vi "CanStatusShow.vi"(10 "DevIndex":u32, 11 "DevType":u16) -> ()   [LabVIEW 2011]
doc: "ID=0x6005"
panel:
  out "label2":string="寄存器信息"
  in  "OK":bool
  out "regTECounter":u8 caption="Send error register:" format="0x%02x"
  out "regRECounter":u8 caption="Receiving error register:" format="0x%02x"
  out "regEWLimit":u8 caption="Error warning limit register:" format="0x%02x"
  out "regECCapture":u8 caption="Error register:" format="0x%02x"
  out "regALCapture":u8 caption="Arbitration lost register:" format="0x%02x"
  out "regStatus":u8 caption="State Register：" format="0x%02x"
  out "regMode":u8 caption="Mode Register:" format="0x%02x"
  out "ErrInterrupt":u8 caption="Interrupt record：" format="0x%02x"
  in  "Update":bool
  in  "udtTime":i32=1 min=1 max=100 format="%d s"
  in  "Auto":bool
  in  "channel":u16(ring) caption="Channel:" items=["Ch1", "Ch2"]
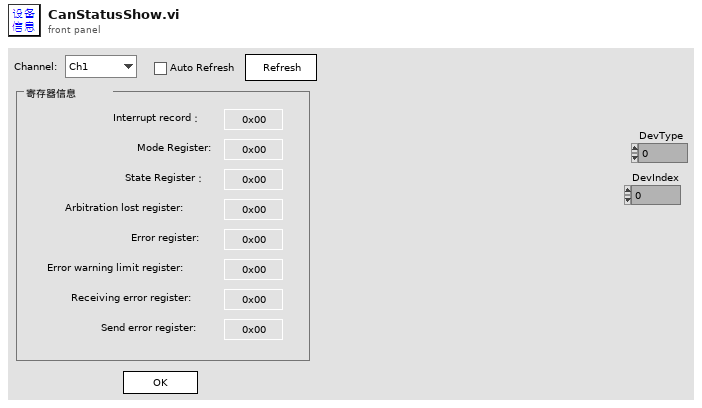
[diagram p1: front panel]
types:
  T1 = cluster{"ErrInterrupt":u8, "regMode":u8, "regStatus":u8, "regALCapture":u8, "regECCapture":u8, "regEWLimit":u8, "regRECounter":u8, "regTECounter":u8, "Reserved":u32}
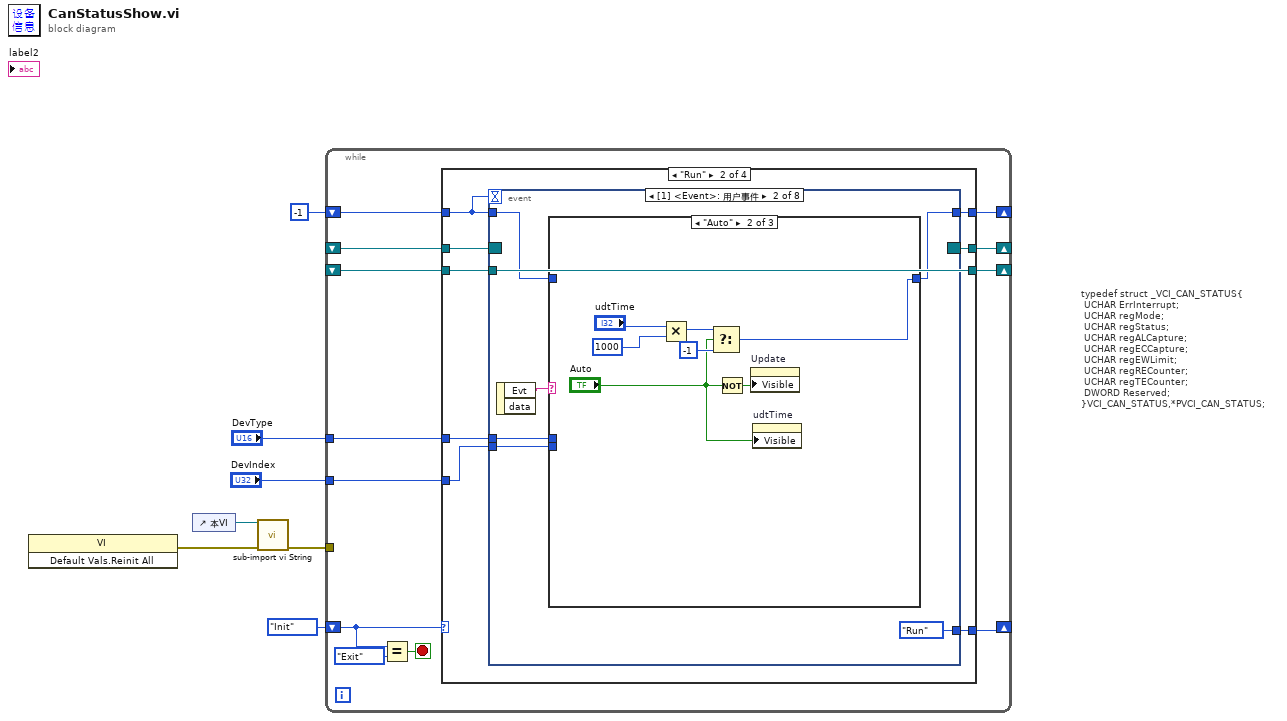
[diagram p0: block diagram]
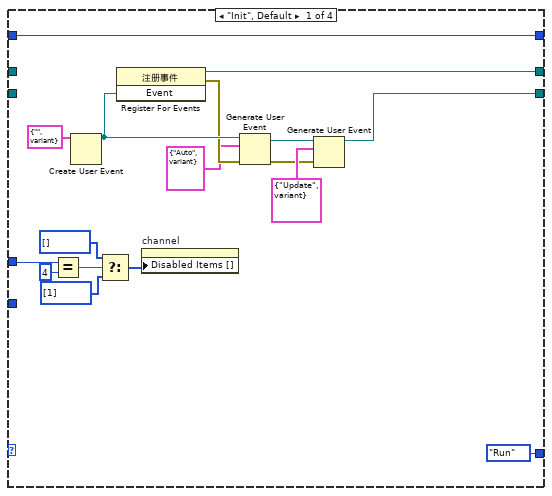
[diagram p2: hidden frame]
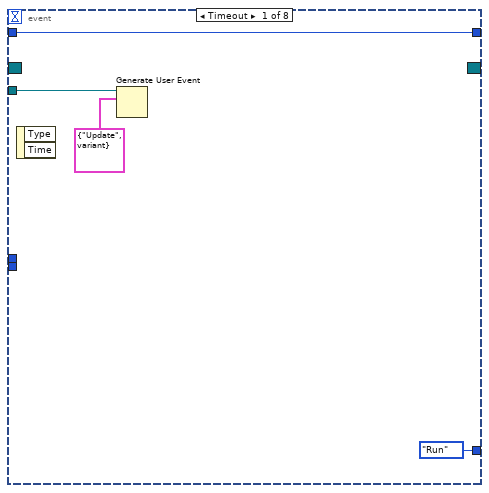
[diagram p3: hidden frame]
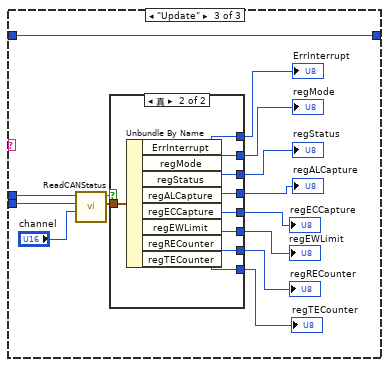
[diagram p5: hidden frame]
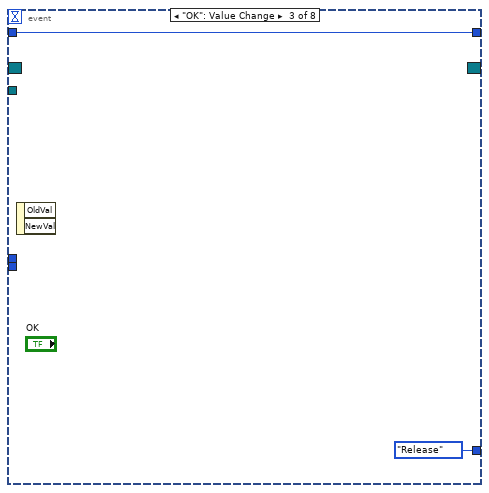
[diagram p7: hidden frame]
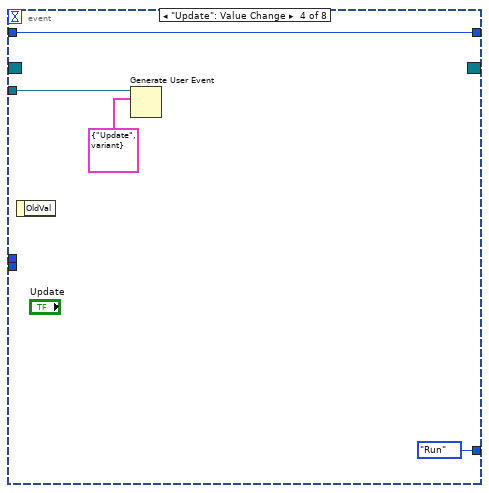
[diagram p8: hidden frame]
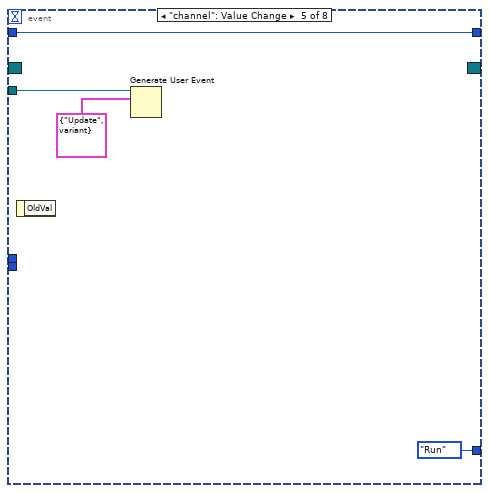
[diagram p9: hidden frame]
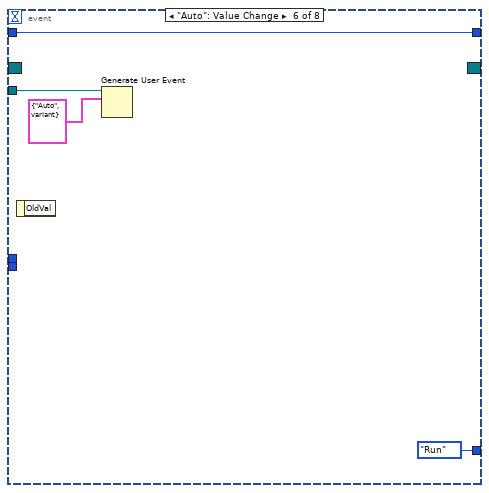
[diagram p10: hidden frame]
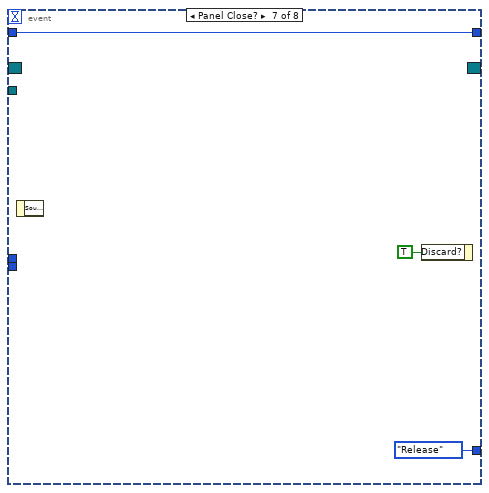
[diagram p11: hidden frame]
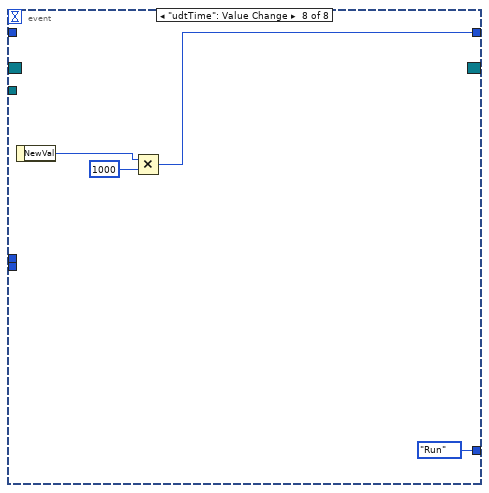
[diagram p12: hidden frame]
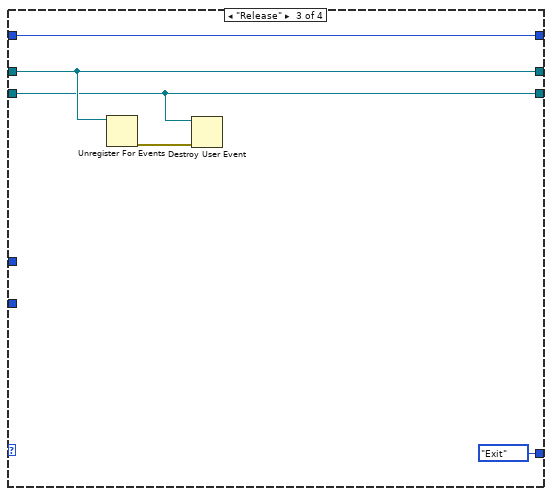
[diagram p13: hidden frame]
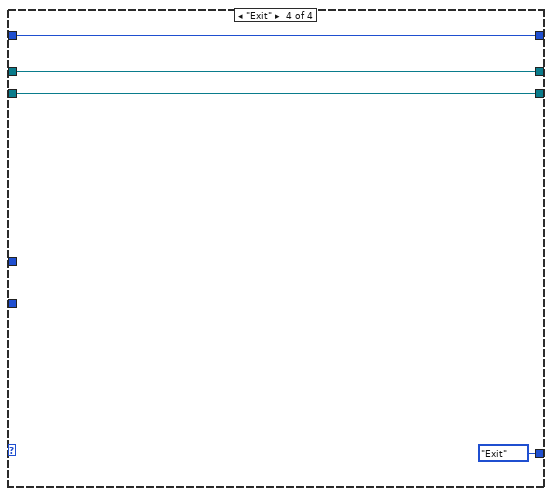
[diagram p14: hidden frame]
diagram:
  # "typedef struct _VCI_CAN_STATUS{\n\tUCHAR\tErrInterrupt;\n\tUCHAR\tregMode;\n\tUCHAR\tregStatus;\n\tUCHAR\tregALCapture;\n\tUCHAR\tregECCapture; \n\tUCHAR\tregEWLimit;\n\tUCHAR\tregRECounter; \n\tUCHAR\tregTECounter;\n\tDWORD\tReserved;\n}VCI_CAN_STATUS,*PVCI_CAN_STATUS;"
  n1 = invoke class="VI" method="Default Vals.Reinit All"() -> (error out=w1:errorcluster)  [unwired: 3 in, 2 out]
  n2 = control-ref of="本VI"() -> (w3:refnum<vi>)
  n3 = call "sub-import vi String.vi"("error in (no error)"=w1, "vi ref"=w3) -> ("error out"=w2:errorcluster)  [unwired: 9 in]
  n4 = while {
    shift-right: [w16] -> _
    shift-left: enum16{"Init", "Run", "Release", "Exit"}."Init" -> [w19]
    shift-right: [w15] -> _
    shift-left: _ -> [w14]
    tunnel: "DevType" -> [w13]
    tunnel: "DevIndex" -> [w12]
    shift-right: [w11] -> _
    shift-left: _ -> [w10]
    shift-right: [w8] -> _
    shift-left: -1 -> [w9]
    tunnel: w2 -> [_]
    stop <- w17 stop-if-true
    n5 = Equal?(x=w19, y=enum16{"Init", "Run", "Release", "Exit"}."Exit") -> (x = y?=w17:bool)
    n6 = case shown="\"Run\"" w19 {
      tunnel: [enum16{"Init", "Run", "Release", "Exit"}."Run" w44 enum16{"Init", "Run", "Release", "Exit"}."Exit" enum16{"Init", "Run", "Release", "Exit"}."Exit"] -> w16
      tunnel: [w34 w42 w110 w115] -> w15
      tunnel: w14 -> [_ w43 w110 w115]
      tunnel: w13 -> [w30 w38 _ _]
      tunnel: w12 -> [_ w37 _ _]
      tunnel: [w21 w41 w109 w114] -> w11
      tunnel: w10 -> [_ w41 w109 w114]
      tunnel: w9 -> [w20 w40 w111 w113]
      tunnel: [w20 w39 w111 w113] -> w8
      frame "Init", Default {
        n7 = Equal?(x=w30, y=u16 4) -> (x = y?=w28:bool)
        n8 = Create User Event(user event datatype=cluster{"Evt":string, "data":variant} {"Evt"="", "data"=variant} ("Event")) -> (user event=w33:refnum<user-event>)  [unwired: 1 in, 1 out]
        n9 = Select(t=i32[] [] ("禁用项[]"), s=w28, f=i32[] [1] ("禁用项[]")) -> (s? t:f=w25:i32[])
        n10 = register-events(w33) -> (reference out=w34:refnum<event-registration>, error out=w32:errorcluster)  [unwired: 2 in]
        n11 = property on="channel" class="Ring (严格)"("Disabled Items []"=w25) -> ()  [unwired: 2 in, 2 out]
        n12 = Generate User Event(user event=w33, event data cluster=cluster{"Evt":string, "data":variant} {"Evt"="Auto", "data"=variant} ("事件数据"), error in=w32) -> (user event out=w23:refnum<user-event>, error out=w22:errorcluster)
        n13 = Generate User Event(user event=w23, event data cluster=cluster{"Evt":string, "data":variant} {"Evt"="Update", "data"=variant} ("事件数据"), error in=w22) -> (user event out=w21:refnum<user-event>)  [unwired: 1 out]
      }
      frame "Run" {
        n14 = event shown="[1] <Event>: 用户事件" {
          selector: w43 -> [_ _ _ _ _ _ _ _]
          dyn-events: [_ _ _ _ _ _ _ _] -> w42
          timeout: w40 -> [_ _ _ _ _ _ _ _]
          tunnel: [enum16{"Init", "Run", "Release", "Exit"}."Run" enum16{"Init", "Run", "Release", "Exit"}."Run" enum16{"Init", "Run", "Release", "Exit"}."Release" enum16{"Init", "Run", "Release", "Exit"}."Run" enum16{"Init", "Run", "Release", "Exit"}."Run" enum16{"Init", "Run", "Release", "Exit"}."Run" enum16{"Init", "Run", "Release", "Exit"}."Release" enum16{"Init", "Run", "Release", "Exit"}."Run"] -> w44
          tunnel: w41 -> [w45 _ _ w88 w92 w98 _ _]
          tunnel: w40 -> [w47 w52 w86 w90 w94 w97 w100 _]
          tunnel: [w47 w51 w86 w90 w94 w97 w100 w103] -> w39
          tunnel: w38 -> [_ w50 _ _ _ _ _ _]
          tunnel: w37 -> [_ w49 _ _ _ _ _ _]
          event Timeout {
            n15 = event-data() -> ()  [unwired: 1 in, 2 out]
            n16 = Generate User Event(user event=w45, event data cluster=cluster{"Evt":string, "data":variant} {"Evt"="Update", "data"=variant} ("事件数据")) -> ()  [unwired: 1 in, 2 out]
          }
          event User Event {
            n17 = event-data() -> ("Evt"=w53:string)  [unwired: 1 in, 1 out]
            n18 = case shown="\"Auto\"" w53 {
              tunnel: w52 -> [w55 _ w76]
              tunnel: [w55 w59 w76] -> w51
              tunnel: w50 -> [_ _ w75]
              tunnel: w49 -> [_ _ w74]
              frame "假", Default {
              }
              frame "Auto" {
                n19 = Multiply(x="udtTime", y=1000) -> (x*y=w60:i32)
                n20 = Select(t=w60, s="Auto", f=-1) -> (s? t:f=w59:i32)
                n21 = Not(x="Auto") -> (.not. x?=w57:bool)
                n22 = property on="Update" class="Bool"("Visible"=w57) -> ()  [unwired: 2 in, 2 out]
                n23 = property on="udtTime" class="DigNum (严格)"("Visible"="Auto") -> ()  [unwired: 2 in, 2 out]
              }
              frame "Update" {
                n24 = call "ReadCANStatus.vi"("CANInd"="channel", "DeciceInd"=w74, "DeviceType"=w75) -> ("VCI_CAN_STATUS"=w71:T1, "Valid"=w72:bool)  [unwired: 6 in, 1 out]
                n25 = case shown="真" w72 {
                  tunnel: w71 -> [_ w85]
                  tunnel: [_ w84] -> w70
                  tunnel: [_ w83] -> w69
                  tunnel: [_ w82] -> w68
                  tunnel: [_ w81] -> w67
                  tunnel: [_ w80] -> w66
                  tunnel: [_ w79] -> w65
                  tunnel: [_ w78] -> w64
                  tunnel: [_ w77] -> w63
                  frame False {
                  }
                  frame True {
                    n26 = Unbundle By Name(w85) -> ("ErrInterrupt"=w84:u8, "regMode"=w83:u8, "regStatus"=w82:u8, "regALCapture"=w81:u8, "regECCapture"=w80:u8, "regEWLimit"=w79:u8, "regRECounter"=w78:u8, "regTECounter"=w77:u8)
                  }
                }
                "ErrInterrupt" <- w70
                "regMode" <- w69
                "regStatus" <- w68
                "regALCapture" <- w67
                "regECCapture" <- w66
                "regEWLimit" <- w65
                "regRECounter" <- w64
                "regTECounter" <- w63
              }
            }
          }
          event "OK": Value Change {
            n27 = event-data() -> ()  [unwired: 1 in, 2 out]
          }
          event "Update": Value Change {
            n28 = event-data() -> ()  [unwired: 1 in, 1 out]
            n29 = Generate User Event(user event=w88, event data cluster=cluster{"Evt":string, "data":variant} {"Evt"="Update", "data"=variant} ("事件数据")) -> ()  [unwired: 1 in, 2 out]
          }
          event "channel": Value Change {
            n30 = event-data() -> ()  [unwired: 1 in, 1 out]
            n31 = Generate User Event(user event=w92, event data cluster=cluster{"Evt":string, "data":variant} {"Evt"="Update", "data"=variant} ("事件数据")) -> ()  [unwired: 1 in, 2 out]
          }
          event "Auto": Value Change {
            n32 = event-data() -> ()  [unwired: 1 in, 1 out]
            n33 = Generate User Event(user event=w98, event data cluster=cluster{"Evt":string, "data":variant} {"Evt"="Auto", "data"=variant} ("事件数据")) -> ()  [unwired: 1 in, 2 out]
          }
          event Panel Close? {
            n34 = event-data() -> ()  [unwired: 1 in, 1 out]
            n35 = event-data("Discard?"=TRUE ("放弃？")) -> ()  [unwired: 1 in, 1 out]
          }
          event "udtTime": Value Change {
            n36 = event-data() -> ("NewVal"=w105:i32)  [unwired: 1 in]
            n37 = Multiply(x=w105, y=1000) -> (x*y=w103:i32)
          }
        }
      }
      frame "Release" {
        n38 = Unregister For Events(event registration refnum=w110) -> (error out=w108:errorcluster)  [unwired: 1 in]
        n39 = Destroy User Event(user event=w109, error in=w108) -> ()  [unwired: 1 out]
      }
      frame "Exit" {
      }
    }
  }
